vi "Convert Kinect Depth Image.vi"(1 "Depth in":dbl[](array[numeric])) -> (0 "Adjust depth out":dbl[](array[numeric]))   [LabVIEW 2010]
uses:
  <vilib>/Analysis/NI_AALPro.lvlib
  <vilib>/Analysis/polynomials.llb/1D Polynomial Evaluation (DBL).vi
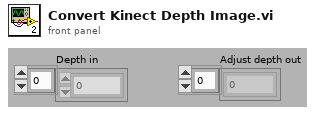
[diagram p1: front panel]
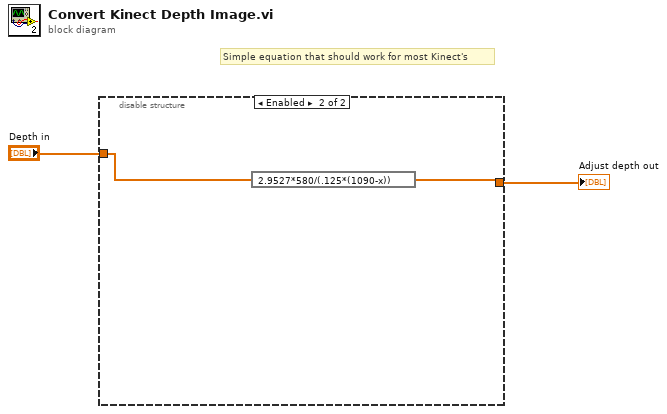
[diagram p0: block diagram]
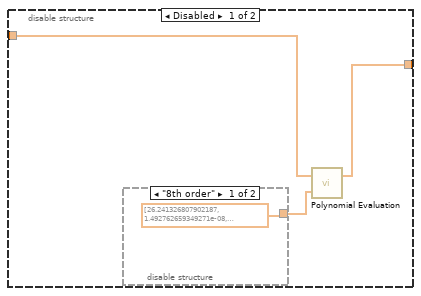
[diagram p2: hidden frame]
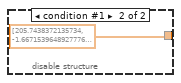
[diagram p3: hidden frame]
diagram:
  # "Simple equation that should work for most Kinect's"
  n1 = disable-structure shown="Enabled" {
    disable-tunnel: [w5 w8] -> w2
    disable-tunnel: "Depth in" -> [w3 w9]
    frame Disabled {
      n2 = disable-structure shown="\"8th order\"" {
        disable-tunnel: [dbl[] [26.241326807902187, 1.492762659349271e-08, 0.00010102880392580251, -5.63883451792149e-06, 3.7404200254627864e-08, -1.0603166551367385e-10, 1.5312182962731e-13, -1.1083923839128109e-16, 3.2003722471423893e-20] ("Polynomial Coefficients") dbl[] [205.7438372135734, -1.6671539648927776, 0.005133550020826422, -6.5549498094181855e-06, 3.027043183851045e-09] ("Polynomial Coefficients")] -> w4
        frame condition #0 (active) {
        }
        frame condition #1 {
        }
      }
      n3 = call-poly <vilib>:"Polynomial Evaluation.vi"("P(x)"=w4, "A"=w3) -> ("P(A)"=w5:dbl[])  [unwired: 1 out]
    }
    frame Enabled {
      n4 = expression code="2.9527*580/(.125*(1090-x))"(w9) -> (w8:dbl[])
    }
  }
  "Adjust depth out" <- w2
